vi "Crosspoint pattern to list.vi"(11 "Pattern":u32[](array[numeric])) -> (3 "List":i32[][](array[numeric]))   [LabVIEW 2020, in "Pickering.lvlib" / "PIPX40 Matrix.lvclass"]
uses:
  PIPX40 Matrix.lvclass
  PIPX40 Matrix.lvclass/PIPX40 Matrix.ctl
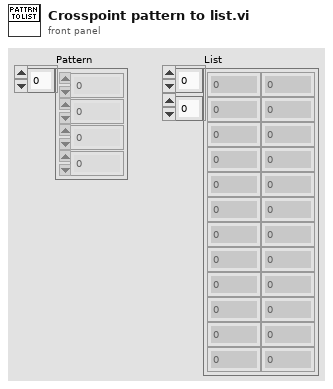
[diagram p1: front panel]
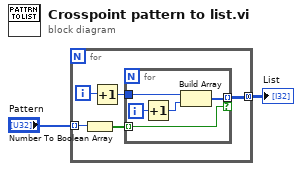
[diagram p0: block diagram]
diagram:
  n1 = for {
    tunnel: "Pattern" -> [w5] mode=indexing
    tunnel: [w4] -> w2 mode=concatenating
    i -> [w7]
    n2 = Number To Boolean Array(number=w5) -> (Boolean array=w3:bool[])
    n3 = Increment(x=w7) -> (x+1=w6:i32)
    n4 = for {
      tunnel: w6 -> [w12]
      tunnel: w3 -> [w8] mode=indexing
      tunnel: [w9] -> w4 mode=indexing if=w8
      i -> [w11]
      n5 = Increment(x=w11) -> (x+1=w10:i32)
      n6 = Build Array(w12, w10) -> (w9:i32[])
    }
  }
  "List" <- w2
